vi "AnalogOut.vi"(8 "error in (no error)":errorcluster, 9 "Existing Obj Name":string, 10 "Pin":string, 11 "mbed_LVLibrary.lvlib:mbed.lvclass":refnum<class "mbed.lvclass">) -> (0 "error out":errorcluster, 1 "Assigned Name":string, 3 "AnalogOut.lvclass 2":refnum<class "AnalogOut.lvclass">)   [LabVIEW 2011, in "mbed_LVLibrary.lvlib" / "AnalogOut.lvclass"]
uses:
  AnalogOut.lvclass
  Transport Mechanisms/mbed/mbed.lvclass
  AnalogOut.lvclass/AnalogOut.ctl
  <vilib>/regexp/Match Regular Expression.xnode
panel:
  in  "AnalogOut.lvclass":refnum<class "AnalogOut.lvclass">
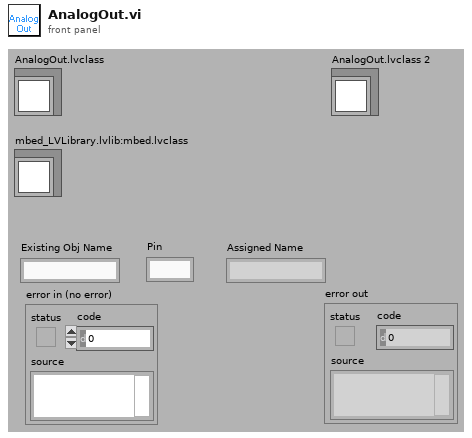
[diagram p1: front panel]
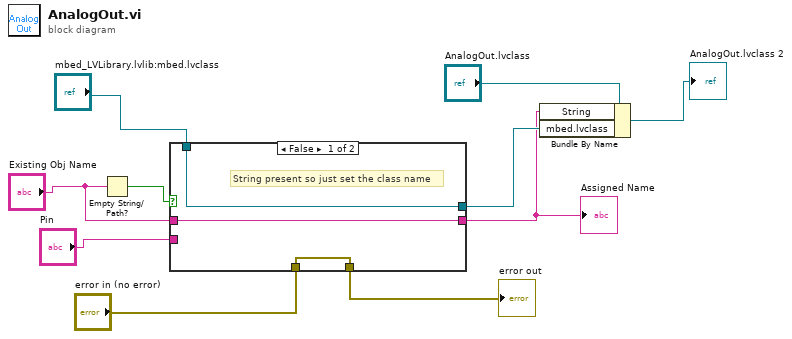
[diagram p0: block diagram]
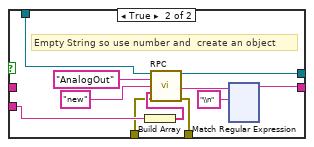
[diagram p2: hidden frame]
diagram:
  n1 = Empty String/Path?(string/path="Existing Obj Name") -> (empty?=w7:bool)
  n2 = case shown="False" w7 {
    tunnel: "Existing Obj Name" -> [w13 _]
    tunnel: [w13 w20] -> w8
    tunnel: "mbed_LVLibrary.lvlib:mbed.lvclass" -> [w12 w24]
    tunnel: [w12 w21] -> w9
    tunnel: "Pin" -> [_ w16]
    tunnel: "error in (no error)" -> [w11 w15]
    tunnel: [w11 w14] -> w2
    frame False {
      # "String present so just set the class name"
    }
    frame True {
      # "Empty String so use number and  create an object"
      n3 = Build Array(w16) -> (w17:string[])
      n4 = call-dynamic "RPC.vi"("mbed in"=w24, "Name"="AnalogOut", "method"="new", "Args"=w17, "error in (no error)"=w15) -> ("mbed out"=w21:refnum<class "mbed.lvclass">, "RPC Result"=w19:string, "error out"=w14:errorcluster)  [unwired: 8 in]
      n5 = xnode "Match Regular Expression"("input string"=w19, "regular expression"="\\n") -> ("before match"=w20:string)  [unwired: 4 in, 4 out]
    }
  }
  "Assigned Name" <- w8
  "error out" <- w2
  n6 = Bundle By Name(cluster="AnalogOut.lvclass", "String"=w8, "mbed.lvclass"=w9) -> (→"AnalogOut.lvclass 2":refnum<class "AnalogOut.lvclass">)
